vi "Load_from_Project.vi"(8 "error in (no error)":errorcluster, 9 "index":i32, 10 "buildObject":T3, 11 "AB_Source_Library in":refnum<class "AB_Source_Library.lvclass">) -> (0 "error out":errorcluster, 2 "linker info":T2, 3 "AB_Source_Library out":refnum<class "AB_Source_Library.lvclass">)   [LabVIEW 2020, in "AB_Source_Library.lvclass"]
uses:
  <vilib>/AppBuilder/AB_Classes/Source/Library/AB_Source_Library.lvclass
  <resource>/Framework/Providers/API/ItemRef.ctl
  <vilib>/Utility/lvfile.llb/LVFileType.ctl
  <vilib>/AppBuilder/RW_Project/AB_RW_Project_PropBag_Action.ctl
  <vilib>/AppBuilder/AB_Classes/Source/Library/AB_Source_Library.lvclass/AB_Source_Library.ctl
  <vilib>/AppBuilder/AB_Classes/Source/AB_Source.lvclass
  <vilib>/Utility/lvfile.llb/NI_FileType.lvlib
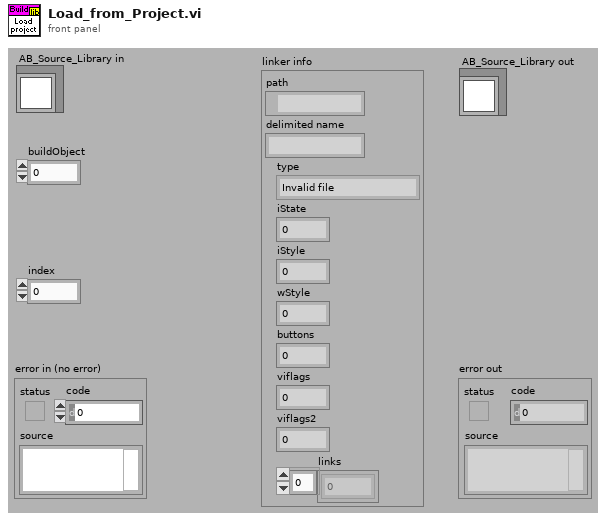
[diagram p1: front panel]
types:
  T1 = typedef "NI_FileType.lvlib/LVFileType.ctl" = enum32{"Invalid file", "Unknown type", "Instrument", "Control", "Polymorphic VI", "Project", "Library", "LVClass", "XControl", "XNode", "Shared library", ".NET assembly", "ActiveX interface", "CIN", "Run-time menu", "Palette menu", "Help file", "LLB", "XNode Edit Dependency", "Class Private Data Control", "Statechart", "MathScript .m file", "Ladder Diagram", "LVLibp", "XNode Build Dependency"}
  T2 = cluster{"path":path, "delimited name":string, "type":T1, "iState":u32, "iStyle":u16, "wStyle":u16, "buttons":u16, "viflags":u32, "viflags2":u32, "links":u32[]}
  T3 = typedef "ItemRef.ctl" = u64
  T4 = typedef "AB_RW_Project_PropBag_Action.ctl" = enum16{"read", "write", "clear", "readPrevious", "writePrevious", "clearPrevious"}
  T5 = typedef "AB_RW_Project_Source_Library_Data.ctl" = cluster{"relinkCallers":bool, "atomicCopy":bool, "allowMissingMembers":bool, "LVLIBPtopLevel":bool}
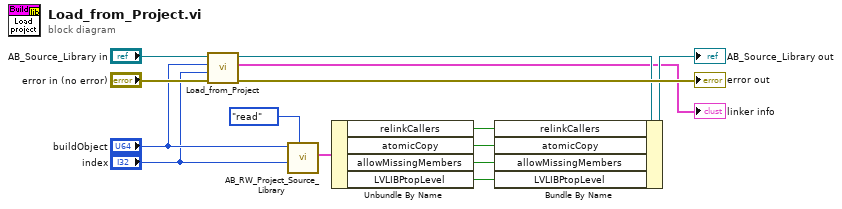
[diagram p0: block diagram]
diagram:
  n1 = call-parent "Load_from_Project.vi"("error in (no error)"="error in (no error)", "index"="index", "buildObject"="buildObject", "AB_Source in"="AB_Source_Library in") -> ("error out"=→"error out":errorcluster, "linker info"=→"linker info":T2, "AB_Source out"=w11:refnum<class "AB_Source_Library.lvclass">)  [unwired: 5 in]
  n2 = call <vilib>:"AB_RW_Project_Source_Library.vi"("action"=AB_RW_Project_PropBag_Action."read", "index in"="index", "buildObject"="buildObject") -> ("dataSource out"=w6:T5)  [unwired: 5 in, 3 out]
  n3 = Unbundle By Name(w6) -> ("relinkCallers"=w5:bool, "atomicCopy"=w4:bool, "allowMissingMembers"=w3:bool, "LVLIBPtopLevel"=w2:bool)
  n4 = Bundle By Name(cluster=w11, "relinkCallers"=w5, "atomicCopy"=w4, "allowMissingMembers"=w3, "LVLIBPtopLevel"=w2) -> (→"AB_Source_Library out":refnum<class "AB_Source_Library.lvclass">)
